vi "Listener Async.vi"(4 "Immutable TLS":refnum<k36>, 6 "TLS":bool, 9 "Listener":refnum<k5>, 10 "Server Endpoint":refnum<class "Endpoint.lvclass">, 11 "Listener Notifier":refnum<notifier>) -> ()   [LabVIEW 2020, in "Stream-Websocket.lvlib" / "Websocket Client.lvclass"]
uses:
  Websocket Client.lvclass
  Listener Result.ctl
  Listener Status.ctl
  C:/dev/lv20CE/relink/lv-stream/stream/Connection/Connection.lvclass
  lv-stream/stream/Endpoint/Endpoint.lvclass
  lv-stream/stream/Connection State.ctl
  lv-stream/stream/URI/URI.lvclass
  Stream-Websocket.lvlib
  lv-stream/stream/Connection/Connection.lvclass
  lv-stream/stream/Stream.lvlib
panel:
  out "URI String":string
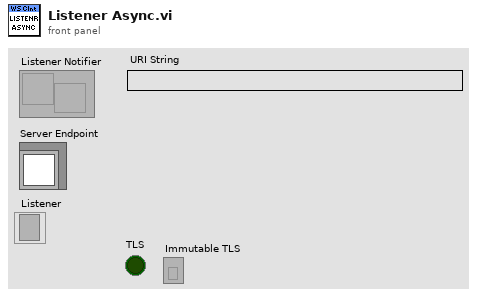
[diagram p1: front panel]
types:
  T1 = typedef "Stream-Websocket.lvlib/Listener Result.ctl" = cluster{"Status":T2, "Client":refnum<class "Websocket Client.lvclass">}
  T2 = typedef "Stream-Websocket.lvlib/Listener Status.ctl" = enum16{"Successful", "Unsuccessful"}
  T3 = typedef "Stream.lvlib/Connection State.ctl" = enum16{"Connected", "Disconnected"}
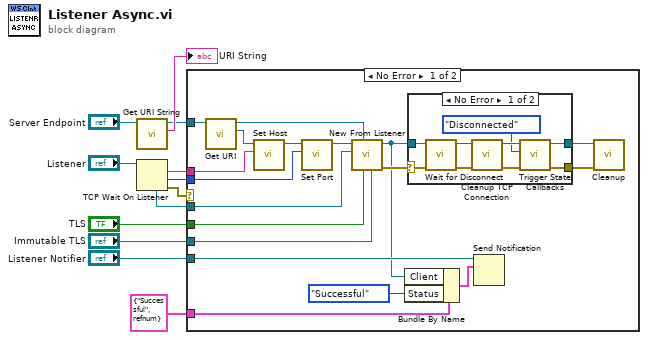
[diagram p0: block diagram]
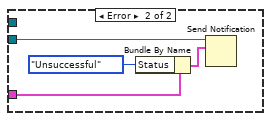
[diagram p3: hidden frame]
diagram:
  n1 = call "Get URI String.vi"("Endpoint in"="Server Endpoint") -> ("URI String"=→"URI String":string, "Endpoint out"=w4:refnum<class "Endpoint.lvclass">)  [unwired: 8 in, 1 out]
  n2 = TCP Wait On Listener(11:"Listener") -> (0:w9:errorcluster, 1:w7:u16, 2:w8:string, 4:w6:refnum<k5>)  [unwired: 3 in, 1 out]
  n3 = case shown="No Error" w9 {
    tunnel: w8 -> [w26 _]
    tunnel: w7 -> [w25 _]
    tunnel: w6 -> [w23 _]
    tunnel: "Listener Notifier" -> [w19 w43]
    tunnel: w4 -> [w27 _]
    tunnel: T1 {"Status"=enum."Successful", "Client"=refnum} ("Listener Result") -> [w21 w45]
    tunnel: "Immutable TLS" -> [w14 _]
    tunnel: "TLS" -> [w13 _]
    frame No Error {
      n4 = call "Get URI.vi"("Endpoint in"=w27) -> ("URI"=w29:refnum<class "URI.lvclass">, "Endpoint out"=w22:refnum<class "Endpoint.lvclass">)  [unwired: 8 in, 1 out]
      n5 = call "Set Host.vi"("Host"=w26, "URI in"=w29) -> ("URI out"=w28:refnum<class "URI.lvclass">)  [unwired: 8 in, 1 out]
      n6 = call "Set Port.vi"("Port"=w25, "URI in"=w28) -> ("URI out"=w24:refnum<class "URI.lvclass">)  [unwired: 8 in, 1 out]
      n7 = call "New From Listener.vi"("Immutable TLS"=w14, "TLS"=w13, "From"=w22, "TCP Connection"=w23, "URI"=w24) -> ("error out"=w30:errorcluster, "Client"=w17:refnum<class "Websocket Client.lvclass">)  [unwired: 5 in]
      n8 = Bundle By Name(cluster=w21, "Client"=w17, "Status"=Listener_Status."Successful") -> (w18:T1)
      n9 = case shown="No Error" w30 {
        selector: w30 -> [w39 w41]
        tunnel: w17 -> [w38 w40]
        tunnel: [w32 w40] -> w16
        tunnel: [w31 w41] -> w15
        frame No Error {
          n10 = call "Wait for Disconnect.vi"("error in (no error)"=w39, "Websocket Client in"=w38) -> ("error out"=w36:errorcluster, "Websocket Client out"=w37:refnum<class "Websocket Client.lvclass">)  [unwired: 8 in]
          n11 = call "Cleanup TCP Connection.vi"("error in (no error)"=w36, "Websocket Client in"=w37) -> ("error out"=w34:errorcluster, "Websocket Client out"=w35:refnum<class "Websocket Client.lvclass">)  [unwired: 8 in]
          n12 = call "Trigger State Callbacks.vi"("error in (no error)"=w34, "State"=Connection_State."Disconnected", "Connection in"=w35) -> ("error out"=w31:errorcluster, "Connection out"=w32:refnum<class "Websocket Client.lvclass">)  [unwired: 7 in]
        }
        frame Error {
        }
      }
      n13 = Send Notification(notification=w18, notifier=w19) -> ()  [unwired: 1 in, 2 out]
      n14 = call-dynamic "Cleanup.vi"("error in (no error)"=w15, "Websocket Client in"=w16) -> ()  [unwired: 9 in, 1 out]
    }
    frame Error {
      n15 = Bundle By Name(cluster=w45, "Status"=Listener_Status."Unsuccessful") -> (w42:T1)
      n16 = Send Notification(notification=w42, notifier=w43) -> ()  [unwired: 1 in, 2 out]
    }
  }
